vi "ftp screenshot.vi"() -> ()   [LabVIEW 2013]
panel:
  in  "path to JPEG file":path=path "D:/Delhi/Shareit/ayodhya-bg.jpg"
  in  "Boolean 3":bool
  in  "Boolean 2":bool
  out "path":path=path "D:/FINALE @25 #bangalore/IMG-20170928-WA0001 - Copy"
  in  "Boolean":bool
  in  "Numeric":dbl
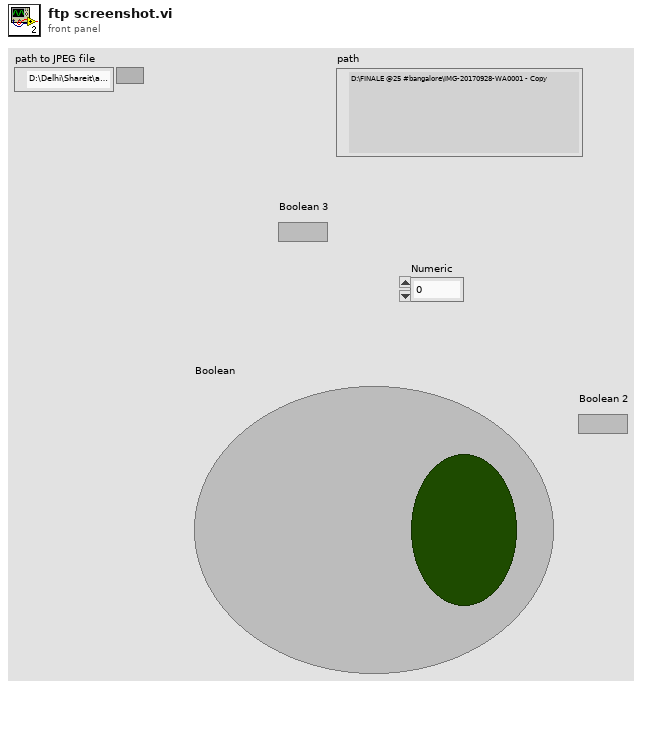
[diagram p1: front panel]
types:
  T1 = typedef "imagedata.ctl" = cluster{"image type":i32, "image depth":i32, "image":u8[], "mask":u8[], "colors":u32[], "Rectangle":cluster{"left":i16, "top":i16, "right":i16, "bottom":i16}}
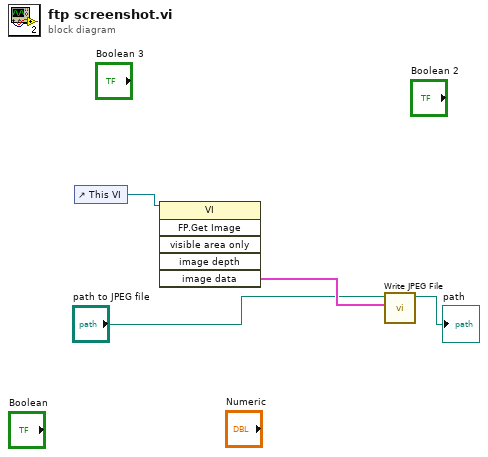
[diagram p0: block diagram]
diagram:
  n1 = control-ref of="This VI"() -> (w3:refnum<vi>)
  n2 = invoke class="VI" method="FP.Get Image"(reference=w3) -> ("image data"=w4:T1)  [unwired: 5 in, 5 out]
  n3 = call <vilib>:"Write JPEG File.vi"("image data"=w4, "path to JPEG file"="path to JPEG file") -> ("path"=→"path":path)  [unwired: 8 in, 1 out]
